vi "U32 to U8s.vi"(2 "U32":u32) -> (15 "HiHi":u8, 16 "Hi":u8, 17 "Lo":u8, 18 "LoLo":u8)   [LabVIEW 2013, in "VRI.lvlib"]
uses:
  VRI.lvlib
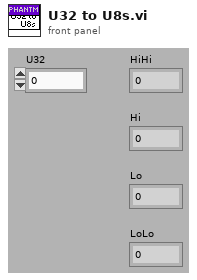
[diagram p1: front panel]
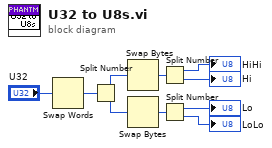
[diagram p0: block diagram]
diagram:
  n1 = Swap Words(1:"U32") -> (0:w5:u32)
  n2 = Split Number(x=w5) -> (hi(x)=w2:u16, lo(x)=w4:u16)
  n3 = Swap Bytes(anything=w2) -> (byte swapped=w1:u16)
  n4 = Swap Bytes(anything=w4) -> (byte swapped=w3:u16)
  n5 = Split Number(x=w1) -> (hi(x)=→"HiHi":u8, lo(x)=→"Hi":u8)
  n6 = Split Number(x=w3) -> (hi(x)=→"Lo":u8, lo(x)=→"LoLo":u8)
